vi "Camera_test.vi"() -> ()   [LabVIEW 2018]
panel:
  out "Image Number":u32
  in  "Number of Image Buffers":u32=10
  in  "Log Image":bool
  out "Frame Rate":dbl
  out "Total Images Transferred":u32
  out "Lost Image Count":u32
  in  "Stop (F)":bool
  out "Image Out":T1(plugin-control)
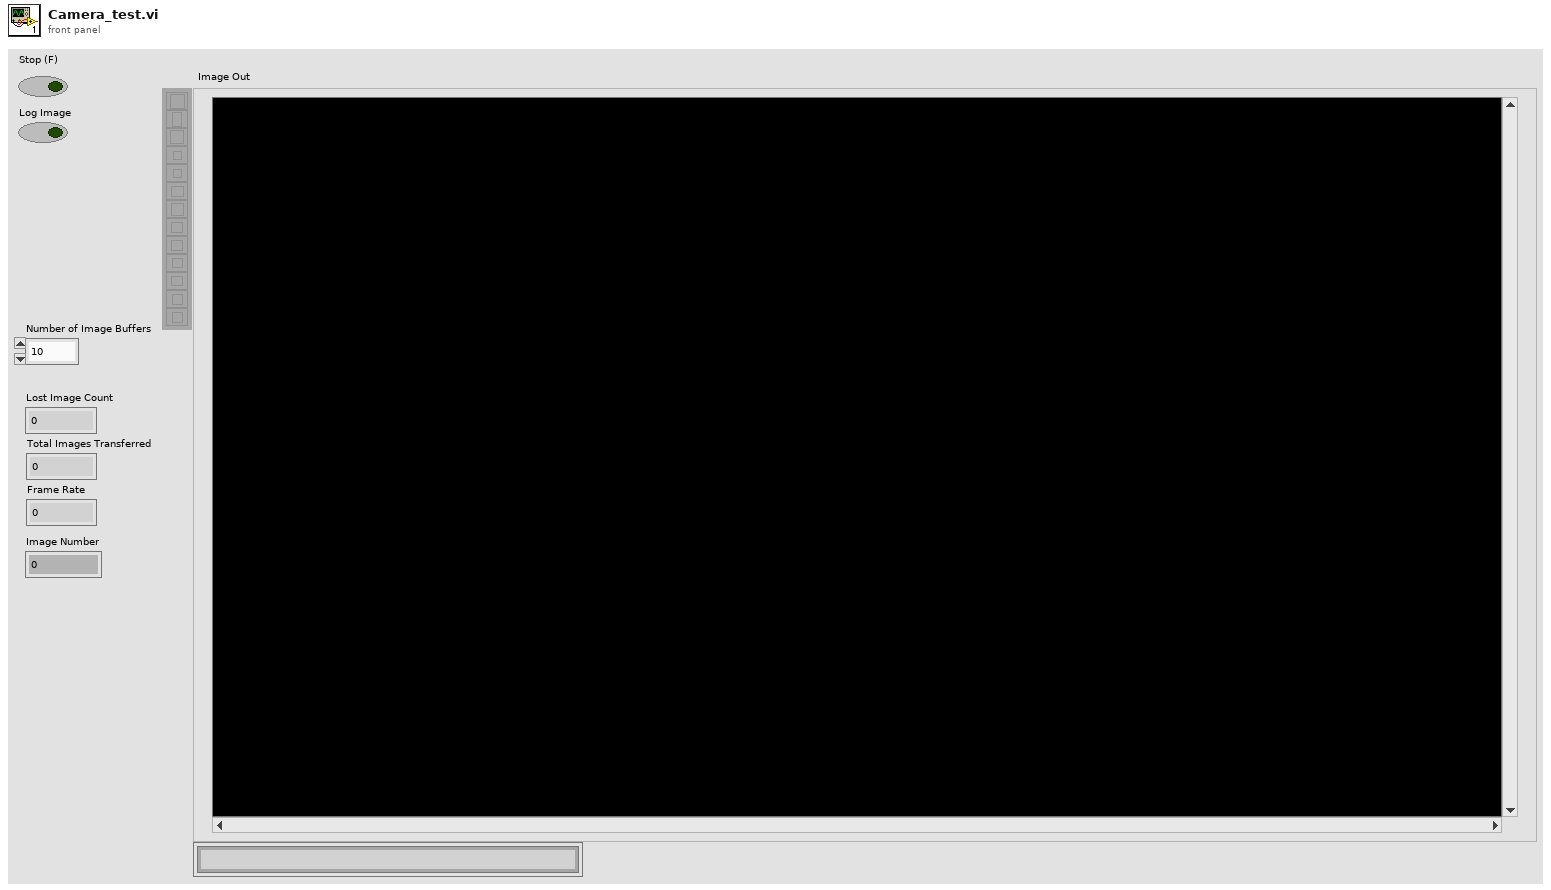
[diagram p1: front panel]
types:
  T1 = typedef "IMAQ Image.ctl" = refnum<image>
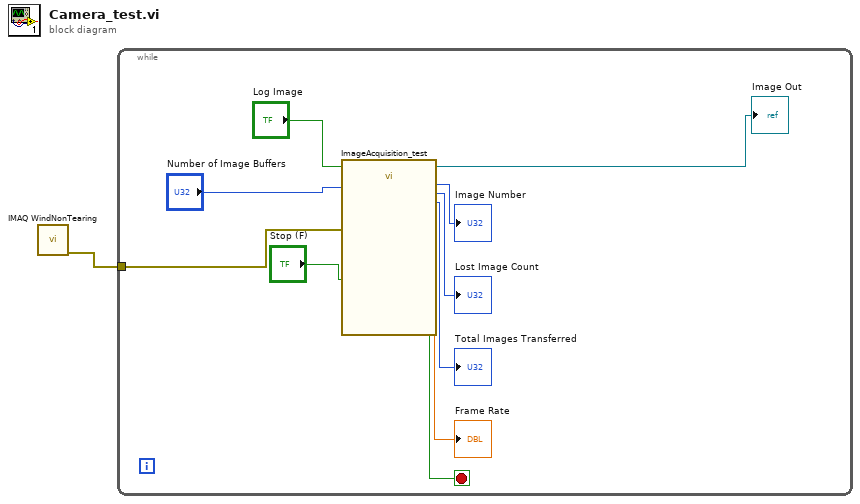
[diagram p0: block diagram]
diagram:
  n1 = call "IMAQ WindNonTearing"() -> ("error out"=w1:errorcluster)  [unwired: 10 in, 1 out]
  n2 = while {
    tunnel: w1 -> [w3]
    stop <- w10 stop-if-true
    n3 = call "ImageAcquisition_test.vi"("Log Image"="Log Image", "Number of Image Buffers"="Number of Image Buffers", "Stop (F)"="Stop (F)", "error in"=w3) -> ("Image Out"=→"Image Out":T1, "Image Number"=→"Image Number":u32, "Lost Image Count"=→"Lost Image Count":u32, "Total Images Transferred"=→"Total Images Transferred":u32, "Frame Rate"=→"Frame Rate":dbl, "Stopped"=w10:bool)  [unwired: 16 in, 2 out]
  }
